vi "get Priority.vi"(11 "Message in":refnum<class "Message.lvclass">) -> (3 "user event priority":T1)   [LabVIEW 2015, in "Message.lvclass"]
uses:
  Message.lvclass
  <vilib>/event_ctls.llb/usereventprio.ctl
  Message.lvclass/Message.ctl
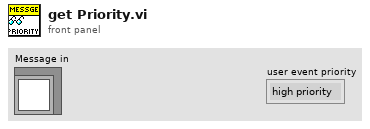
[diagram p1: front panel]
types:
  T1 = typedef "usereventprio.ctl" = enum32{"high priority", "normal priority"}
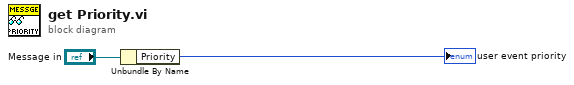
[diagram p0: block diagram]
diagram:
  n1 = Unbundle By Name("Message in") -> ("Priority"=→"user event priority":T1)
